vi "ReadRingBlock_SD.vi"(1 "pixel":u32=1, 2 "stop":i32, 3 "start":i32=1) -> (0 "Data Values":u32[][](graph))   [LabVIEW 2015]
uses:
  DLL/ESLSCDLL.dll
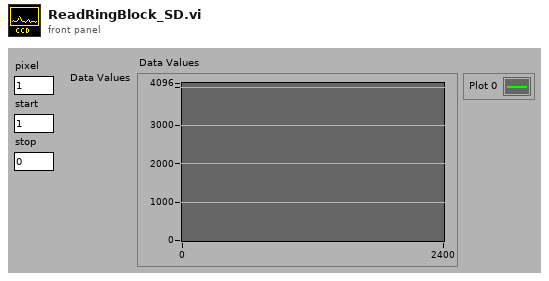
[diagram p1: front panel]
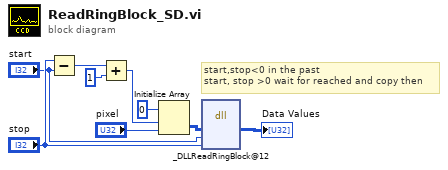
[diagram p0: block diagram]
diagram:
  # "start,stop<0 in the past\nstart, stop >0 wait for reached and copy then"
  n1 = Subtract(x="stop", y="start") -> (x-y=w5:i32)
  n2 = Add(x=w5, y=1) -> (x+y=w4:i32)
  n3 = Initialize Array(u32 0, w4, "pixel") -> (w7:u32[][])
  n4 = dll-call lib="G:/SD/TRANCON-2015/DLL/ESLSCDLL.dll" fn="_DLLReadRingBlock@12" ("lwlscdll.dll:DLLReadLoop")("dioden"=w7, "start"="start", "stop"="stop") -> ("dioden"=→"Data Values":u32[][])  [unwired: 6 in, 2 out]
